vi "Read Configuration (INI) File.vi"() -> (1 "HS INI data":T1, 2 "TC INI data":T3, 3 "V/C INI data":T2)   [LabVIEW 2025]
doc: "Illustrates how to read a configuration settings file. Run Write Configuration (INI) File.vi. Then run this VI."
uses:
  <vilib>/Utility/config.llb/Read Key (Boolean).vi
  <vilib>/Utility/config.llb/Read Key (Double).vi
  <vilib>/Utility/config.llb/Read Key (Path).vi
  <vilib>/Utility/config.llb/Read Key (String).vi
  <vilib>/Utility/config.llb/Read Key (I32).vi
  <vilib>/Utility/config.llb/NI_LVConfig.lvlib
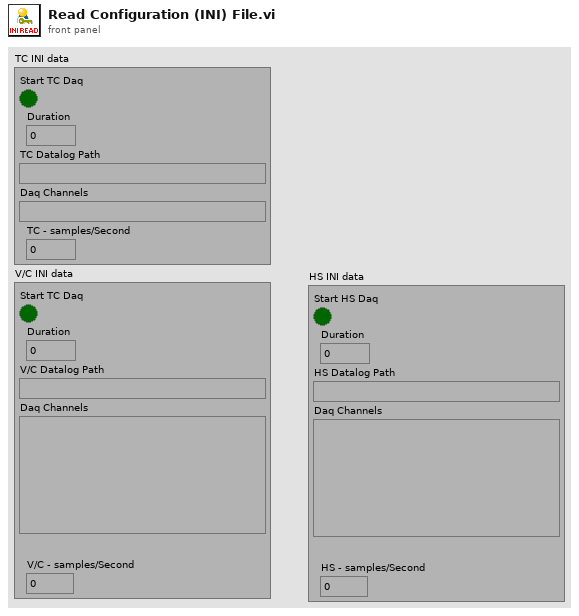
[diagram p1: front panel]
types:
  T1 = cluster{"Start HS Daq":bool, "Duration":dbl, "HS Datalog Path":path, "Daq Channels":string, "HS - samples/Second":i32}
  T2 = cluster{"Start TC Daq":bool, "Duration":dbl, "V/C Datalog Path":path, "Daq Channels":string, "V/C - samples/Second":i32}
  T3 = cluster{"Start TC Daq":bool, "Duration":dbl, "TC Datalog Path":path, "Daq Channels":string, "TC - samples/Second":i32}
  T4 = typedef "NI_LVConfig.lvlib/Config Data RefNum.ctl" = refnum<k1>
  T5 = cluster{"value":bool, "value":dbl, "value":path, "value":string, "value":i32}
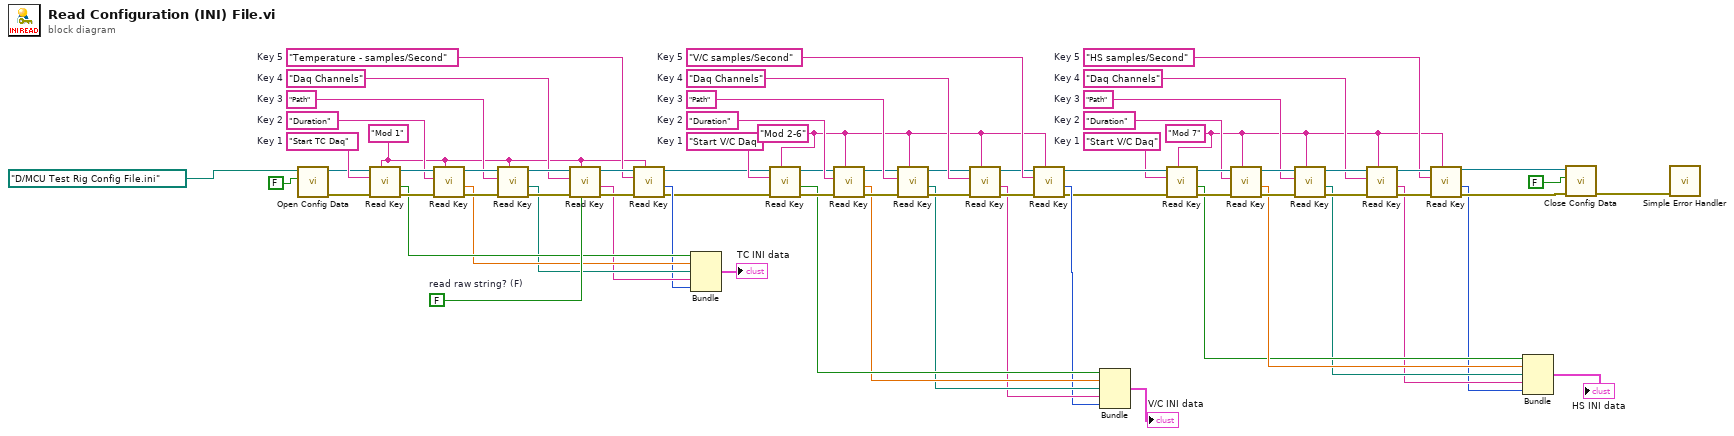
[diagram p0: block diagram]
diagram:
  w10 = "HS samples/Second"  # Key 5
  w11 = "Daq Channels"  # Key 4
  w12 = "Path"  # Key 3
  w13 = "Duration"  # Key 2
  w14 = "Start V/C Daq"  # Key 1
  w7 = "Mod 7" ("section")
  w46 = "V/C samples/Second"  # Key 5
  w45 = "Daq Channels"  # Key 4
  w44 = "Path"  # Key 3
  w43 = "Duration"  # Key 2
  w42 = "Start V/C Daq"  # Key 1
  w23 = "Mod 2-6" ("section")
  w56 = FALSE  # read raw string? (F)
  w61 = "Temperature - samples/Second"  # Key 5
  w62 = "Daq Channels"  # Key 4
  w63 = "Path"  # Key 3
  w64 = "Duration"  # Key 2
  w65 = "Start TC Daq"  # Key 1
  w54 = "Mod 1" ("section")
  n1 = call <vilib>:"Open Config Data.vi"("create file if necessary (T)"=FALSE ("create file if necessary? (T)"), "configuration file path"=path "D:/MCU Test Rig Config File.ini" ("default name")) -> ("error out"=w60:errorcluster, "refnum"=w59:T4)  [unwired: 7 in, 1 out]
  n2 = call-poly <vilib>:"Read Key.vi"("section"=w54, "error in (no error)"=w60, "key"=w65, "refnum"=w59) -> ("error out"=w73:errorcluster, "value"=w52:bool, "refnum out"=w71:T4)  [unwired: 1 in, 4 out]
  n3 = call-poly <vilib>:"Read Key.vi"("section"=w54, "error in (no error)"=w73, "key"=w64, "refnum"=w71) -> ("error out"=w68:errorcluster, "value"=w51:dbl, "refnum out"=w69:T4)  [unwired: 1 in, 4 out]
  n4 = call-poly <vilib>:"Read Key.vi"("section"=w54, "error in (no error)"=w68, "key"=w63, "refnum"=w69) -> ("error out"=w72:errorcluster, "value"=w50:path, "refnum out"=w70:T4)  [unwired: 1 in, 4 out]
  n5 = call-poly <vilib>:"Read Key.vi"("read raw string? (F)"=w56, "section"=w54, "error in (no error)"=w72, "key"=w62, "refnum"=w70) -> ("error out"=w67:errorcluster, "value"=w49:string, "refnum out"=w66:T4)  [unwired: 1 in, 3 out]
  n6 = call-poly <vilib>:"Read Key.vi"("section"=w54, "error in (no error)"=w67, "key"=w61, "refnum"=w66) -> ("error out"=w32:errorcluster, "value"=w48:i32, "refnum out"=w33:T4)  [unwired: 2 in, 3 out]
  n7 = Bundle("value"=w52, "value"=w51, "value"=w50, "value"=w49, "value"=w48) -> (→"TC INI data":T5)  [unwired: 1 in]
  n8 = call-poly <vilib>:"Read Key.vi"("section"=w23, "error in (no error)"=w32, "key"=w42, "refnum"=w33) -> ("error out"=w34:errorcluster, "value"=w31:bool, "refnum out"=w36:T4)  [unwired: 1 in, 4 out]
  n9 = call-poly <vilib>:"Read Key.vi"("section"=w23, "error in (no error)"=w34, "key"=w43, "refnum"=w36) -> ("error out"=w39:errorcluster, "value"=w30:dbl, "refnum out"=w38:T4)  [unwired: 1 in, 4 out]
  n10 = call-poly <vilib>:"Read Key.vi"("section"=w23, "error in (no error)"=w39, "key"=w44, "refnum"=w38) -> ("error out"=w35:errorcluster, "value"=w29:path, "refnum out"=w37:T4)  [unwired: 1 in, 4 out]
  n11 = call-poly <vilib>:"Read Key.vi"("section"=w23, "error in (no error)"=w35, "key"=w45, "refnum"=w37) -> ("error out"=w40:errorcluster, "value"=w28:string, "refnum out"=w41:T4)  [unwired: 2 in, 3 out]
  n12 = call-poly <vilib>:"Read Key.vi"("section"=w23, "error in (no error)"=w40, "key"=w46, "refnum"=w41) -> ("error out"=w25:errorcluster, "value"=w27:i32, "refnum out"=w26:T4)  [unwired: 2 in, 3 out]
  n13 = Bundle("value"=w31, "value"=w30, "value"=w29, "value"=w28, "value"=w27) -> (→"V/C INI data":T5)  [unwired: 1 in]
  n14 = call-poly <vilib>:"Read Key.vi"("section"=w7, "error in (no error)"=w25, "key"=w14, "refnum"=w26) -> ("error out"=w22:errorcluster, "value"=w5:bool, "refnum out"=w20:T4)  [unwired: 1 in, 4 out]
  n15 = call-poly <vilib>:"Read Key.vi"("section"=w7, "error in (no error)"=w22, "key"=w13, "refnum"=w20) -> ("error out"=w17:errorcluster, "value"=w6:dbl, "refnum out"=w18:T4)  [unwired: 1 in, 4 out]
  n16 = call-poly <vilib>:"Read Key.vi"("section"=w7, "error in (no error)"=w17, "key"=w12, "refnum"=w18) -> ("error out"=w21:errorcluster, "value"=w4:path, "refnum out"=w19:T4)  [unwired: 1 in, 4 out]
  n17 = call-poly <vilib>:"Read Key.vi"("section"=w7, "error in (no error)"=w21, "key"=w11, "refnum"=w19) -> ("error out"=w16:errorcluster, "value"=w3:string, "refnum out"=w15:T4)  [unwired: 2 in, 3 out]
  n18 = call-poly <vilib>:"Read Key.vi"("section"=w7, "error in (no error)"=w16, "key"=w10, "refnum"=w15) -> ("error out"=w9:errorcluster, "value"=w2:i32, "refnum out"=w8:T4)  [unwired: 2 in, 3 out]
  n19 = Bundle("value"=w5, "value"=w6, "value"=w4, "value"=w3, "value"=w2) -> (→"HS INI data":T5)  [unwired: 1 in]
  n20 = call <vilib>:"Close Config Data.vi"("error in (no error)"=w9, "write file if changed (T)"=FALSE ("write configuration file? (T)"), "refnum"=w8) -> ("error out"=w55:errorcluster)  [unwired: 8 out]
  n21 = call <vilib>:"Simple Error Handler.vi"("error in (no error)"=w55) -> ()  [unwired: 1 in, 8 out]
